vi "ukol4.vi"() -> ()   [LabVIEW 2023]
uses:
  <vilib>/Analysis/2dsp.llb/Integral Method.ctl
  <vilib>/Analysis/NI_AALPro.lvlib
panel:
  out "Waveform Graph 3":waveform(dbl)[](graph)
  out "Waveform Graph 2":waveform(dbl)[](graph)
  out "Waveform Graph":waveform(dbl)(graph)
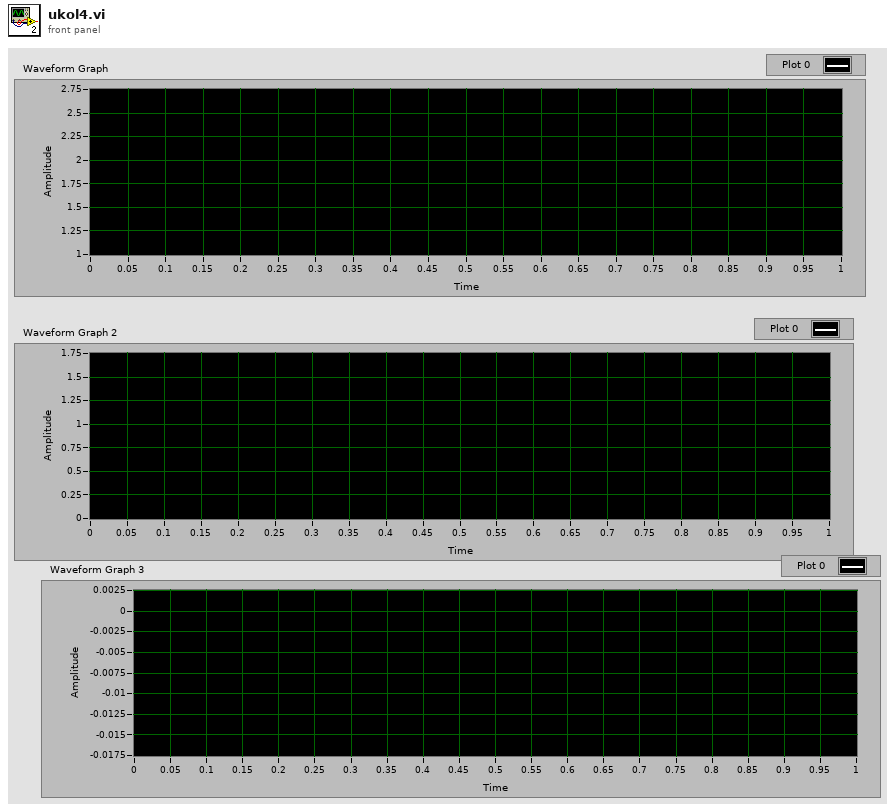
[diagram p1: front panel]
types:
  T1 = typedef "NI_AALPro.lvlib/Integral Method.ctl" = i32
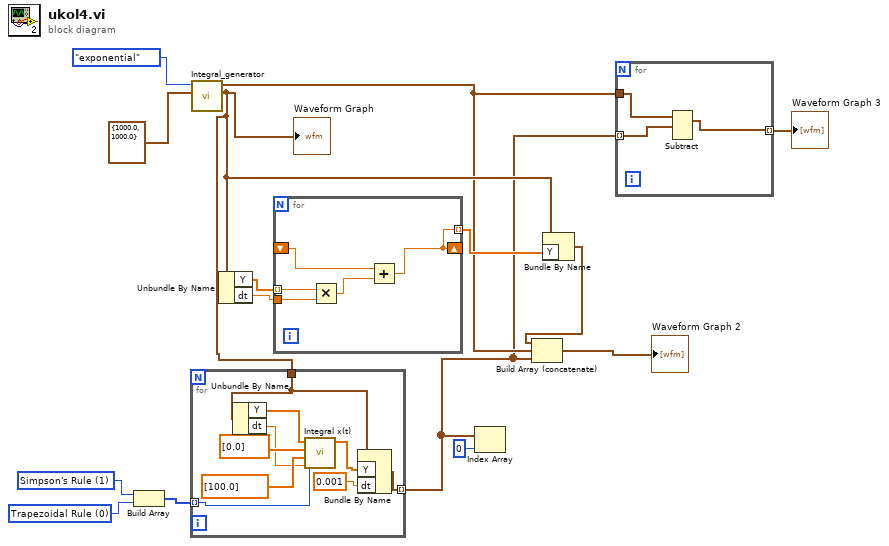
[diagram p0: block diagram]
diagram:
  w11 = T1 0 items=["Trapezoidal Rule", "Simpson's Rule", "Simpson's 3/8 Rule", "Bode Rule"] ("integration method")
  w12 = T1 1 items=["Trapezoidal Rule", "Simpson's Rule", "Simpson's 3/8 Rule", "Bode Rule"] ("integration method")
  n1 = Build Array(w12, w11) -> (w13:T1[])
  n2 = call "Integral_generator.vi"("sampling info"=cluster{"Fs":dbl, "#s":dbl} {"Fs"=1000.0, "#s"=1000.0}, "Signal Type"=enum16{"sine", "polynom", "exponential"}."exponential") -> ("Signal out"=w7:waveform(dbl), "integral out"=w2:waveform(dbl))  [unwired: 7 in, 1 out]
  "Waveform Graph" <- w7
  n3 = for {
    tunnel: w13 -> [w19] mode=indexing
    tunnel: [w23] -> w1 mode=indexing
    tunnel: w7 -> [w16]
    n4 = Unbundle By Name(w16) -> ("Y"=w18:dbl[], "dt"=w17:dbl)
    n5 = call <vilib>:"Integral x(t).vi"("integration method"=w19, "dt"=w17, "Final Condition"=dbl[] [100.0], "Initial Condition"=dbl[] [0.0], "X"=w18) -> ("Integral X"=w22:dbl[])  [unwired: 5 in, 1 out]
    n6 = Bundle By Name(cluster=w16, "Y"=w22, "dt"=0.001) -> (w23:waveform(dbl))
  }
  n7 = Unbundle By Name(w7) -> ("Y"=w9:dbl[], "dt"=w5:dbl)
  n8 = for {
    shift-right: [w25] -> _
    shift-left: _ -> [w26]
    tunnel: w9 -> [w29] mode=indexing
    tunnel: [w25] -> w8 mode=indexing
    tunnel: w5 -> [w28]
    n9 = Multiply(x=w29, y=w28) -> (x*y=w27:dbl)
    n10 = Add(x=w26, y=w27) -> (x+y=w25:dbl)
  }
  n11 = Index Array(array=w1, index=0) -> ()  [unwired: 1 out]
  n12 = Bundle By Name(cluster=w7, "Y"=w8) -> (w6:waveform(dbl))
  n13 = Build Array (concatenate)(w6, w2, w1) -> (→"Waveform Graph 2":waveform(dbl)[])
  n14 = for {
    tunnel: [w32] -> w3 mode=indexing
    tunnel: w2 -> [w31]
    tunnel: w1 -> [w30] mode=indexing
    n15 = Subtract(1:w30, 2:w31) -> (0:w32:waveform(dbl))  [unwired: 1 in, 1 out]
  }
  "Waveform Graph 3" <- w3
